vi "IMG_PARAMS - GetDataFormat.vi"(8 "error in (no error)":errorcluster, 11 "xiApi.NET.ImgParams":refnum<k24>) -> (0 "error out":errorcluster, 3 "xiApi.NET.ImgParams Out":refnum<k24>, 4 "DataFormat":i32, 6 "IMG_FORMAT":T1=enum."RAW16")   [LabVIEW 2013]
doc: "Returns data format of the last acquired image."
uses:
  C:/Projects/Cameras3.x/xiLib/xiLIB_64bit/xiLIB/xiCamLib/API/x64/xiApi.NETX64.dll
  xiLIB_64bit/xiLIB/xiCamLib/API/x64/xiApi.NETX64.dll
  IMG_FORMAT/IMG_DATA_FORMAT.ctl
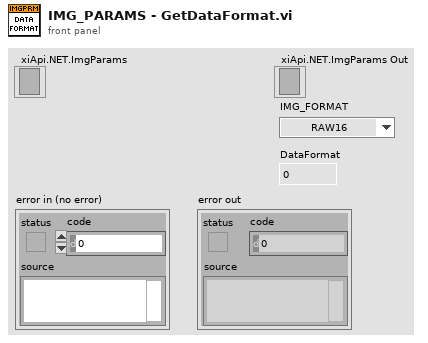
[diagram p1: front panel]
types:
  T1 = typedef "IMG_DATA_FORMAT.ctl" = enum16{"MONO8", "MONO16", "RGB24", "RGB32", "RGBPLANAR", "RAW8", "RAW16"}
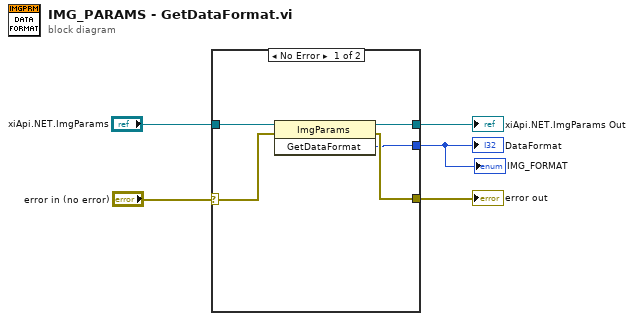
[diagram p0: block diagram]
diagram:
  n1 = case shown="No Error" "error in (no error)" {
    selector: "error in (no error)" -> [w8 w11]
    tunnel: "xiApi.NET.ImgParams" -> [w10 w12]
    tunnel: [w9 w12] -> w4
    tunnel: [w7 w11] -> w2
    tunnel: [w6 _] -> w1
    frame No Error {
      n2 = invoke class="ImgParams" method="GetDataFormat"(reference=w10, error in=w8) -> (reference out=w9:refnum<k24>, error out=w7:errorcluster, "GetDataFormat"=w6:i32)  [unwired: 1 in]
    }
    frame Error {
    }
  }
  "xiApi.NET.ImgParams Out" <- w4
  "error out" <- w2
  "DataFormat" <- w1
  "IMG_FORMAT" <- w1
